vi "test_DisallowedCharsInName_CheckPluginNameIsValid_NameInvalid.vi"() -> (6 "pass":bool, 8 "result":string, 15 "error out":errorcluster)   [LabVIEW 2021]
uses:
  <vilib>/ErrorRing/Error Ring.xnode
  Generator/_Editor/Generator Helpers.lvlib
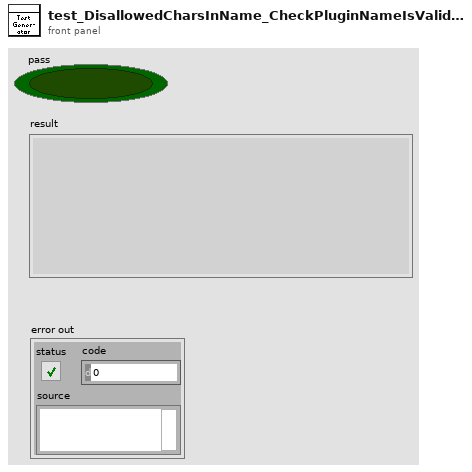
[diagram p1: front panel]
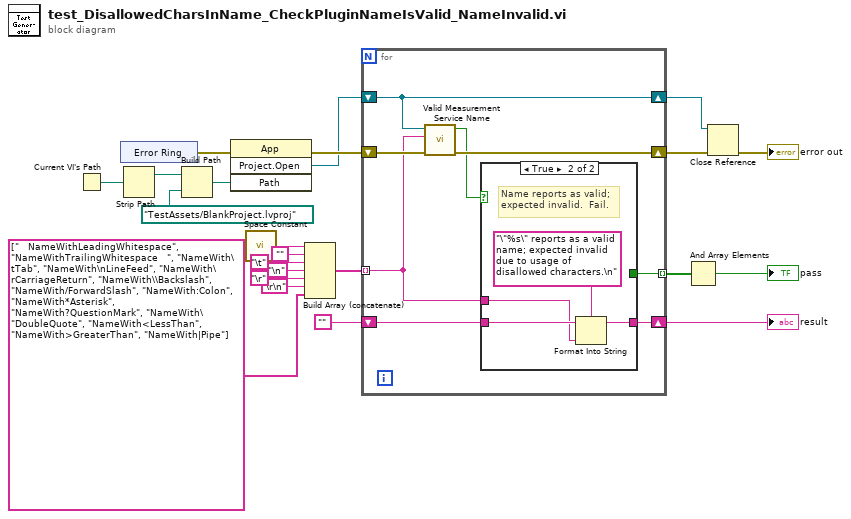
[diagram p0: block diagram]
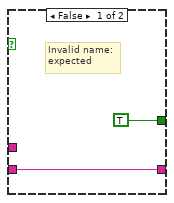
[diagram p2: hidden frame]
diagram:
  n1 = Current VI's Path() -> (path=w22:path)
  n2 = xnode "Error Ring"() -> ("error out"=w19:errorcluster)
  n3 = Strip Path(path=w22) -> (stripped path=w21:path)  [unwired: 1 out]
  n4 = Build Path(base path=w21, name or relative path=path "TestAssets/BlankProject.lvproj" ("path")) -> (appended path=w18:path)
  n5 = invoke class="App" method="Project.Open"(error in=w19, "Path"=w18) -> (error out=w10:errorcluster, "Project:Open"=w9:refnum<vi>)  [unwired: 2 in, 2 out]
  n6 = call <vilib>:"Space Constant.vi"() -> ("String"=w6:string)
  n7 = Build Array (concatenate)(w6, "" ("EmptyString"), "\t" ("Tab Constant"), "\n" ("Line Feed Constant"), "\r", "\r\n", string[] ["   NameWithLeadingWhitespace", "NameWithTrailingWhitespace   ", "NameWith\tTab", "NameWith\nLineFeed", "NameWith\rCarriageReturn", "NameWith\\Backslash", "NameWith/ForwardSlash", "NameWith:Colon", "NameWith*Asterisk", "NameWith?QuestionMark", "NameWith\"DoubleQuote", "NameWith<LessThan", "NameWith>GreaterThan", "NameWith|Pipe"]) -> (w1:string[])
  n8 = for {
    shift-right: [w29] -> w17
    shift-left: w10 -> [w30]
    tunnel: w1 -> [w23] mode=indexing
    shift-right: [w28] -> w15
    shift-left: w9 -> [w28]
    shift-right: [w25] -> w13
    shift-left: "" -> [w26]
    tunnel: [w24] -> w12 mode=indexing
    n9 = call "Valid Measurement Service Name.vi"("error in"=w30, "requested plugin name"=w23, "project ref"=w28) -> ("error out"=w29:errorcluster, "valid name?"=w27:bool)  [unwired: 7 in]
    n10 = case shown="True" w27 {
      tunnel: w26 -> [w32 w36]
      tunnel: [w32 w35] -> w25
      tunnel: [TRUE _] -> w24
      tunnel: w23 -> [_ w34]
      frame False {
        # "Invalid name:\nexpected"
      }
      frame True {
        # "Name reports as valid;\nexpected invalid.  Fail."
        n11 = Format Into String(format string="\"%s\" reports as a valid name; expected invalid due to usage of disallowed characters.\n", initial string=w36, w34) -> (resulting string=w35:string)  [unwired: 1 in, 1 out]
      }
    }
  }
  "result" <- w13
  n12 = And Array Elements(Boolean array=w12) -> (logical AND=→"pass":bool)
  n13 = Close Reference(reference=w15, error in (no error)=w17) -> (error out=→"error out":errorcluster)
